vi "Convert R to Rotation Vector rvec (Rodrigues).vi"() -> ()   [LabVIEW 2025]
uses:
  <vilib>/Analysis/Matrix/Datatypes/RealMatrix.ctl
  <vilib>/gmath/NumericalOptimization/LM model function reference.ctl
  <vilib>/gmath/NumericalOptimization/Nonlinear Curve Fit LM.vi
  <vilib>/gmath/NI_Gmath.lvlib
  <vilib>/Analysis/Matrix/NI_Matrix.lvlib
panel:
  out "covariance":dbl[][][](array[numeric])
  out "best fit parameters":dbl[][](array[numeric])
  out "best nonlinear fit":dbl[][](array[numeric])
  out "Array":i32[](array[numeric])
  in  "t Translation Vector":dbl[](array[numeric])
  in  "R Rotation Matrix":T1 format="%#_6f"
  in  "Measured Points":dbl[][](array[numeric])
  in  "World corner points (out)":dbl[][](array[numeric])=[[-3.25, -3.25, 0.0], [3.25, -3.25, 0.0], [3.25, 3.25, 0.0], [-3.25, 3.25, 0.0]]
  in  "cy height":dbl format="%.5f"
  in  "cx width":dbl format="%.5f"
  in  "f_px":dbl format="%.5f"
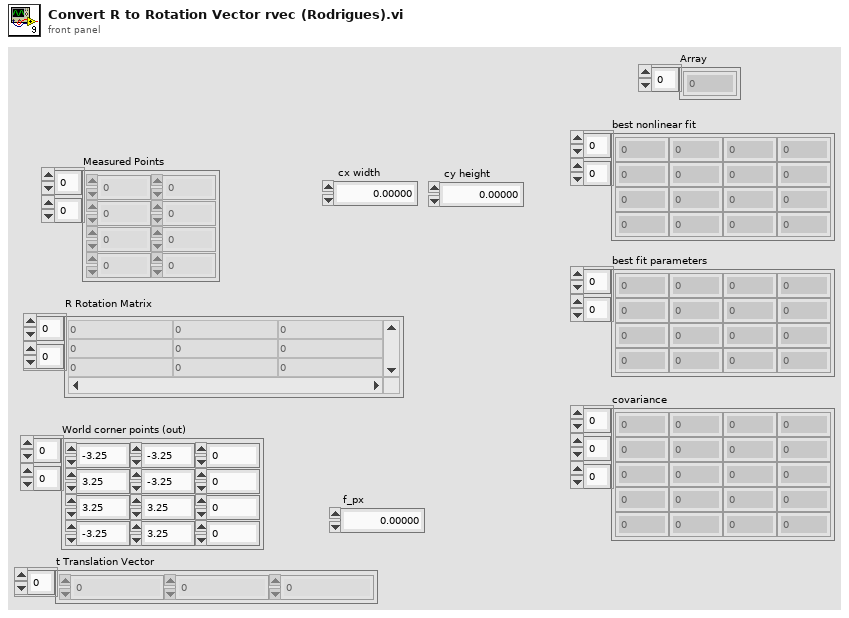
[diagram p1: front panel]
types:
  T1 = typedef "NI_Matrix.lvlib/RealMatrix.ctl" = dbl[][]
  T2 = typedef "NI_Gmath.lvlib/LM model function reference.ctl" = refnum<vi>
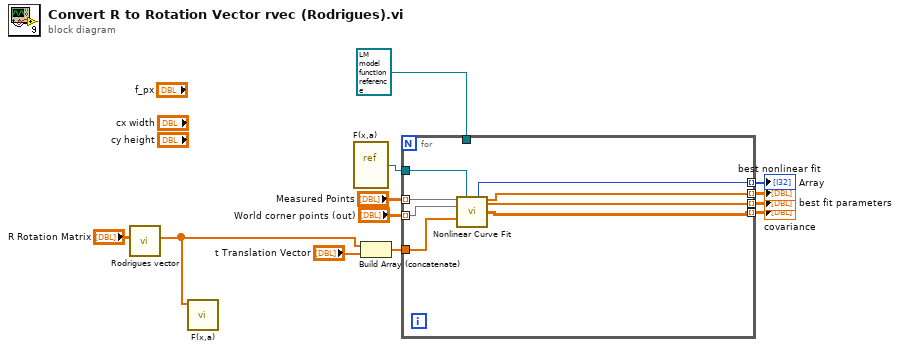
[diagram p0: block diagram]
diagram:
  n1 = call "Rodrigues vector.vi"("R Rotation Matrix"="R Rotation Matrix") -> ("Rodrigues vector"=w1:dbl[])  [unwired: 10 in]
  n2 = call "F(x,a).vi"("a"=w1) -> ()  [unwired: 3 in, 3 out]
  n3 = vi-ref "F(x,a).vi"() -> (w2:refnum<vi>)
  n4 = Build Array (concatenate)(w1, "t Translation Vector") -> (w9:dbl[])
  n5 = for {
    tunnel: "Measured Points" -> [w20] mode=indexing
    tunnel: "World corner points (out)" -> [w19] mode=indexing
    tunnel: w9 -> [w18]
    tunnel: [w17] -> w6 mode=indexing
    tunnel: [w16] -> w5 mode=indexing
    tunnel: [w15] -> w4 mode=indexing
    tunnel: [w14] -> w7 mode=indexing
    tunnel: T2 refnum ("f(x,a)") -> [_]
    tunnel: w2 -> [w13]
    n6 = call-poly <vilib>:"Nonlinear Curve Fit.vi"("Y"=w20, "f(x,a)"=w13, "X"=w19, "initial parameters"=w18) -> ("number of function calls"=w14:i32, "best nonlinear fit"=w17:dbl[], "best fit parameters"=w16:dbl[], "covariance"=w15:T1)  [unwired: 6 in, 2 out]
  }
  "Array" <- w7
  "best nonlinear fit" <- w6
  "best fit parameters" <- w5
  "covariance" <- w4
